vi "Socket Monitor.vi"(7 "path override":path, 8 "error in (no error)":errorcluster, 9 "events_":i32, 10 "addr_":string, 11 "s_":u32) -> (0 "error out":errorcluster, 2 "function return":i32, 3 "s_ out":u32)   [LabVIEW 2025, in "LibZMQ.lvlib"]
doc: "ZMQ_EXPORT int zmq_socket_monitor (void *s_, const char *addr_, int events_);"
uses:
  LibZMQ.lvlib
  errno.vi
  strerror.vi
  <vilib>/Utility/error.llb/Error Cluster From Error Code.vi
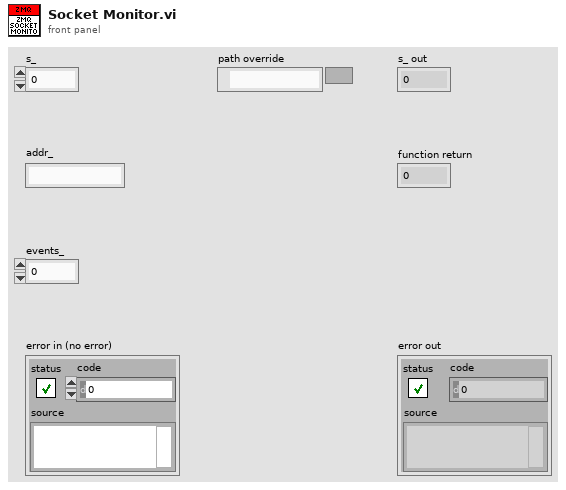
[diagram p1: front panel]
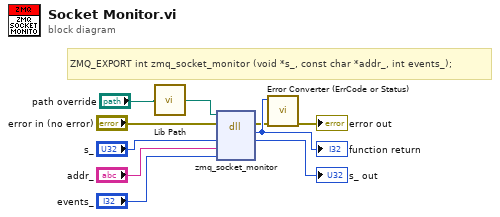
[diagram p0: block diagram]
diagram:
  # "ZMQ_EXPORT int zmq_socket_monitor (void *s_, const char *addr_, int events_);"
  n1 = call "Lib Path.vi"("path override"="path override") -> ("lib path"=w2:path)
  n2 = dll-call lib="C:/git/ZA/libzmq-v143-mt-4_3_6/lib/win32/libzmq-v143-mt-4_3_6.dll" fn="zmq_socket_monitor"(path in=w2, error in="error in (no error)", "s_"="s_", "addr_"="addr_", "events_"="events_") -> (error out=w4:errorcluster, "return type"=w10:i32, "s_"=→"s_ out":u32)  [unwired: 3 in, 1 out]
  "function return" <- w10
  n3 = call "Error Converter (ErrCode or Status).vi"("error in (no error)"=w4, "error code"=w10) -> ("error out"=→"error out":errorcluster)  [unwired: 9 in]
